vi "HexU16_to_DecString.vi"(5 "String":string="0f 23", 7 "offset (0)":i32) -> (6 "decimal integer string":string, 8 "number":u32)   [LabVIEW 2018]
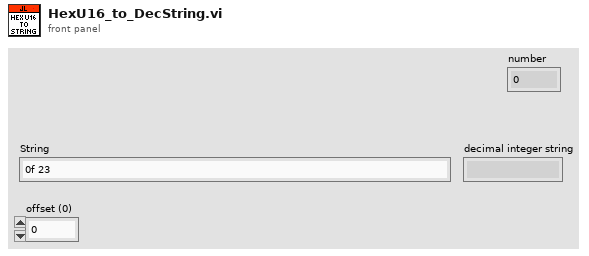
[diagram p1: front panel]
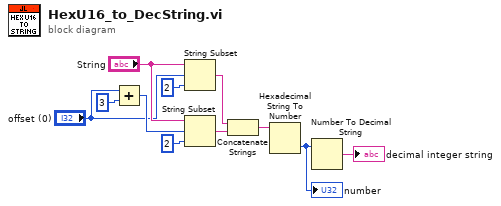
[diagram p0: block diagram]
diagram:
  n1 = Add(x="offset (0)", y=3) -> (x+y=w3:i32)
  n2 = String Subset(string="String", offset (0)="offset (0)", length (rest)=2 ("offset (0)")) -> (substring=w9:string)
  n3 = String Subset(string="String", offset (0)=w3, length (rest)=2 ("length (rest)")) -> (substring=w8:string)
  n4 = Concatenate Strings(w9, w8) -> (w6:string)
  n5 = Hexadecimal String To Number(string=w6) -> (number=w5:u32)  [unwired: 2 in, 1 out]
  "number" <- w5
  n6 = Number To Decimal String(number=w5) -> (decimal integer string=→"decimal integer string":string)  [unwired: 1 in]
